vi "Generador_DAQ_Demanda.vi"() -> ()   [LabVIEW 2015]
uses:
  <vilib>/DAQmx/write.llb/DAQmx Write (Analog DBL 1Chan 1Samp).vi
  <vilib>/DAQmx/create/channels.llb/DAQmx Create Channel (AO-Voltage-Basic).vi
  <vilib>/DAQmx/miscellaneous.llb/DAQmx Fill In Error Info.vi
panel:
  in  "Knob":dbl(knob) scale=0.0..10.0
  in  "stop":bool
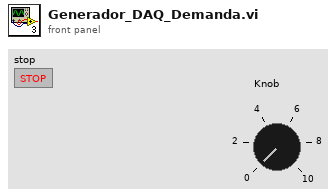
[diagram p1: front panel]
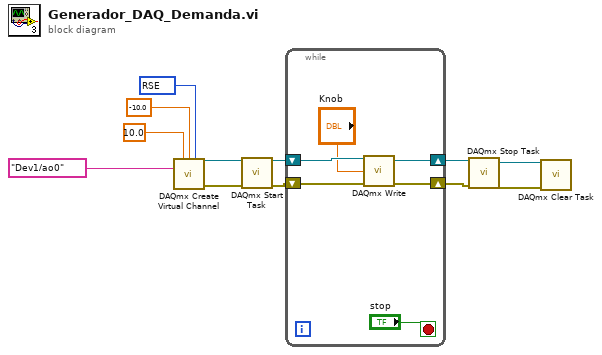
[diagram p0: block diagram]
diagram:
  w12 = 10083 items=["Default"=-1, "RSE"=10083, "Differential"=10106, "Pseudodifferential"=12529] ("output terminal configuration")
  n1 = call-poly <vilib>:"DAQmx Create Virtual Channel.vi"("maximum value"=10.0, "minimum value"=-10.0, "output terminal configuration"=w12, "physical channels"=tag "Dev1/ao0") -> ("task out"=w2:refnum<k21>, "error out"=w1:errorcluster)  [unwired: 10 in]
  n2 = call <vilib>:"DAQmx Start Task.vi"("task/channels in"=w2, "error in"=w1) -> ("task out"=w6:refnum<k21>, "error out"=w5:errorcluster)  [unwired: 12 in]
  n3 = while {
    shift-right: [w16] -> w4
    shift-left: w6 -> [w18]
    shift-right: [w15] -> w3
    shift-left: w5 -> [w17]
    stop <- "stop" stop-if-true
    n4 = call-poly <vilib>:"DAQmx Write.vi"("task/channels in"=w18, "data"="Knob", "error in"=w17) -> ("task out"=w16:refnum<k21>, "error out"=w15:errorcluster)  [unwired: 10 in, 1 out]
  }
  n5 = call <vilib>:"DAQmx Stop Task.vi"("task/channels in"=w4, "error in"=w3) -> ("task out"=w8:refnum<k21>, "error out"=w7:errorcluster)  [unwired: 12 in]
  n6 = call <vilib>:"DAQmx Clear Task.vi"("task in"=w8, "error in"=w7) -> ()  [unwired: 13 in, 1 out]
